vi "Get Available Engine Sim Components.vi"(10 "Register info":T16) -> (2 "Engine Sim Components":T1)   [LabVIEW 2011, in "Engine Sim System Explorer.lvlib"]
uses:
  Engine Sim System Explorer.lvlib
  <userlib>/_FPGA Interface Advanced Tools/FPGA Bitfile Utility/TypeDefs/Scalar Register Set.ctl
  <userlib>/_FPGA Interface Advanced Tools/FPGA Bitfile Utility/TypeDefs/Scalar Register.ctl
  <userlib>/_FPGA Interface Advanced Tools/FPGA Bitfile Utility/TypeDefs/Array Register Set.ctl
  <userlib>/_FPGA Interface Advanced Tools/FPGA Bitfile Utility/TypeDefs/Array Register.ctl
  <userlib>/_FPGA Interface Advanced Tools/FPGA Bitfile Utility/TypeDefs/FIFO Channel Set.ctl
  <userlib>/_FPGA Interface Advanced Tools/FPGA Bitfile Utility/TypeDefs/FIFO Channel.ctl
  TypeDefs/EngineSimComps.ctl
  TypeDefs/APUComp.ctl
  TypeDefs/NTeethComp.ctl
  TypeDefs/FullyCustomComp.ctl
  Shared/FullyCustomCommMode.ctl
  TypeDefs/FullyCustomProfilesComp.ctl
  TypeDefs/ECUEventComp.ctl
  TypeDefs/DataReplayLoopComp.ctl
  TypeDefs/DataReplayComp.ctl
  Engine Simulation Shared.lvlib
  <userlib>/_FPGA Interface Advanced Tools/FPGA Bitfile Utility/FPGA Bitfile Utility.lvlib
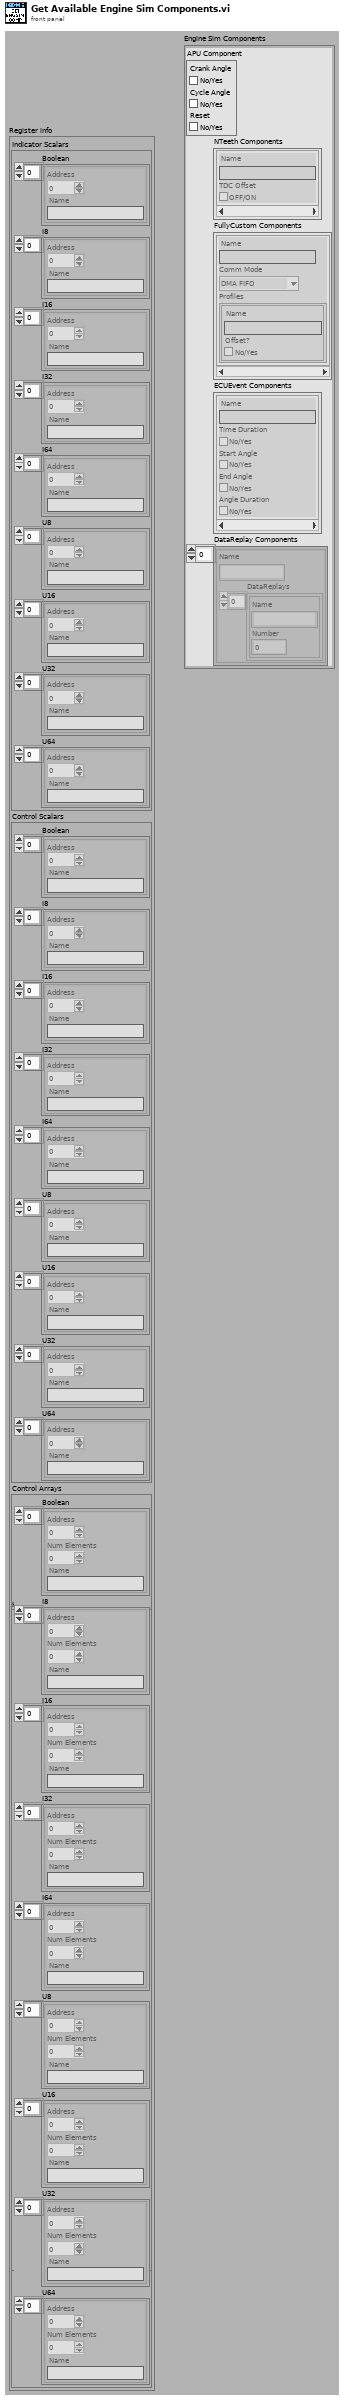
[diagram p1: front panel]
types:
  T1 = typedef "Engine Sim System Explorer.lvlib/EngineSimComps.ctl" = cluster{"APU Component":T2, "NTeeth Components":T3[], "FullyCustom Components":T4[], "ECUEvent Components":T7[], "DataReplay Components":T8[]}
  T2 = typedef "Engine Sim System Explorer.lvlib/APUComp.ctl" = cluster{"Crank Angle":bool, "Cycle Angle":bool, "Reset":bool}
  T3 = typedef "Engine Sim System Explorer.lvlib/NTeethComp.ctl" = cluster{"Name":string, "TDC Offset":bool}
  T4 = typedef "Engine Sim System Explorer.lvlib/FullyCustomComp.ctl" = cluster{"Name":string, "Comm Mode":T5, "Profiles":T6[]}
  T5 = typedef "Engine Simulation Shared.lvlib/FullyCustomCommMode.ctl" = enum16{"DMA FIFO", "FP Data Transfer"}
  T6 = typedef "Engine Sim System Explorer.lvlib/FullyCustomProfilesComp.ctl" = cluster{"Name":string, "Offset?":bool}
  T7 = typedef "Engine Sim System Explorer.lvlib/ECUEventComp.ctl" = cluster{"Name":string, "Time Duration":bool, "Start Angle":bool, "End Angle":bool, "Angle Duration":bool}
  T8 = typedef "Engine Sim System Explorer.lvlib/DataReplayLoopComp.ctl" = cluster{"Name":string, "DataReplays":T9[]}
  T9 = typedef "Engine Sim System Explorer.lvlib/DataReplayComp.ctl" = cluster{"Name":string, "Number":u8}
  T10 = typedef "FPGA Bitfile Utility.lvlib/Scalar Register Set.ctl" = cluster{"Boolean":T11[], "I8":T11[], "I16":T11[], "I32":T11[], "I64":T11[], "U8":T11[], "U16":T11[], "U32":T11[], "U64":T11[]}
  T11 = typedef "FPGA Bitfile Utility.lvlib/Scalar Register.ctl" = cluster{"Address":u32, "Name":string}
  T12 = typedef "FPGA Bitfile Utility.lvlib/Array Register Set.ctl" = cluster{"Boolean":T13[], "I8":T13[], "I16":T13[], "I32":T13[], "I64":T13[], "U8":T13[], "U16":T13[], "U32":T13[], "U64":T13[]}
  T13 = typedef "FPGA Bitfile Utility.lvlib/Array Register.ctl" = cluster{"Address":u32, "Num Elements":u32, "Name":string}
  T14 = typedef "FPGA Bitfile Utility.lvlib/FIFO Channel Set.ctl" = cluster{"Boolean":T15[], "I8":T15[], "I16":T15[], "I32":T15[], "I64":T15[], "U8":T15[], "U16":T15[], "U32":T15[], "U64":T15[]}
  T15 = typedef "FPGA Bitfile Utility.lvlib/FIFO Channel.ctl" = cluster{"Physical Channel":u32, "Name":string}
  T16 = cluster{"Indicator Scalars":T10, "Control Scalars":T10, "Control Arrays":T12, "HostToTarget":T14}
  T17 = cluster{cluster{"Name":string, "Offset":bool}[]}[]
  T18 = typedef "Engine Sim System Explorer.lvlib/FullyCustomRegs.ctl" = cluster{"Num Angles":bool, "Num Profiles":bool, "Angles FIFO":bool, "Data":bool, "Toggle":bool, "LoadComplete":bool, "Profiles":cluster{"First Rising?":bool, "Offset":bool}[]}
  T19 = cluster{"FullyCustomTeeth Names":string[], "FullyCustomTeeths Profile Names":cluster{"FullyCustomTeeth Profile Names":string[]}[], "FullyCustomTeeth Regs":T18[]}
  T20 = typedef "Engine Sim System Explorer.lvlib/ECUEventRegs.ctl" = cluster{"Time Duration":bool, "Start Angle":bool, "End Angle":bool, "Angle Duration":bool}
  T21 = cluster{"ECUEvent Names":string[], "ECUEvent Regs":T20[]}
  T22 = typedef "Engine Sim System Explorer.lvlib/NTeethRegs.ctl" = cluster{"Deg High Pulse":bool, "Deg Low Pulse":bool, "TDC High?":bool, "Num Teeth Miss":bool, "Miss Teeth Offset":bool, "TDC Offset":bool}
  T23 = cluster{"NTeeth Names":string[], "NTeeth Regs":T22[]}
  T24 = cluster{"FullyCustomTeeth Profile Names":string[]}[]
  T25 = cluster{"FullyCustomTeeth Profile Names":string[]}
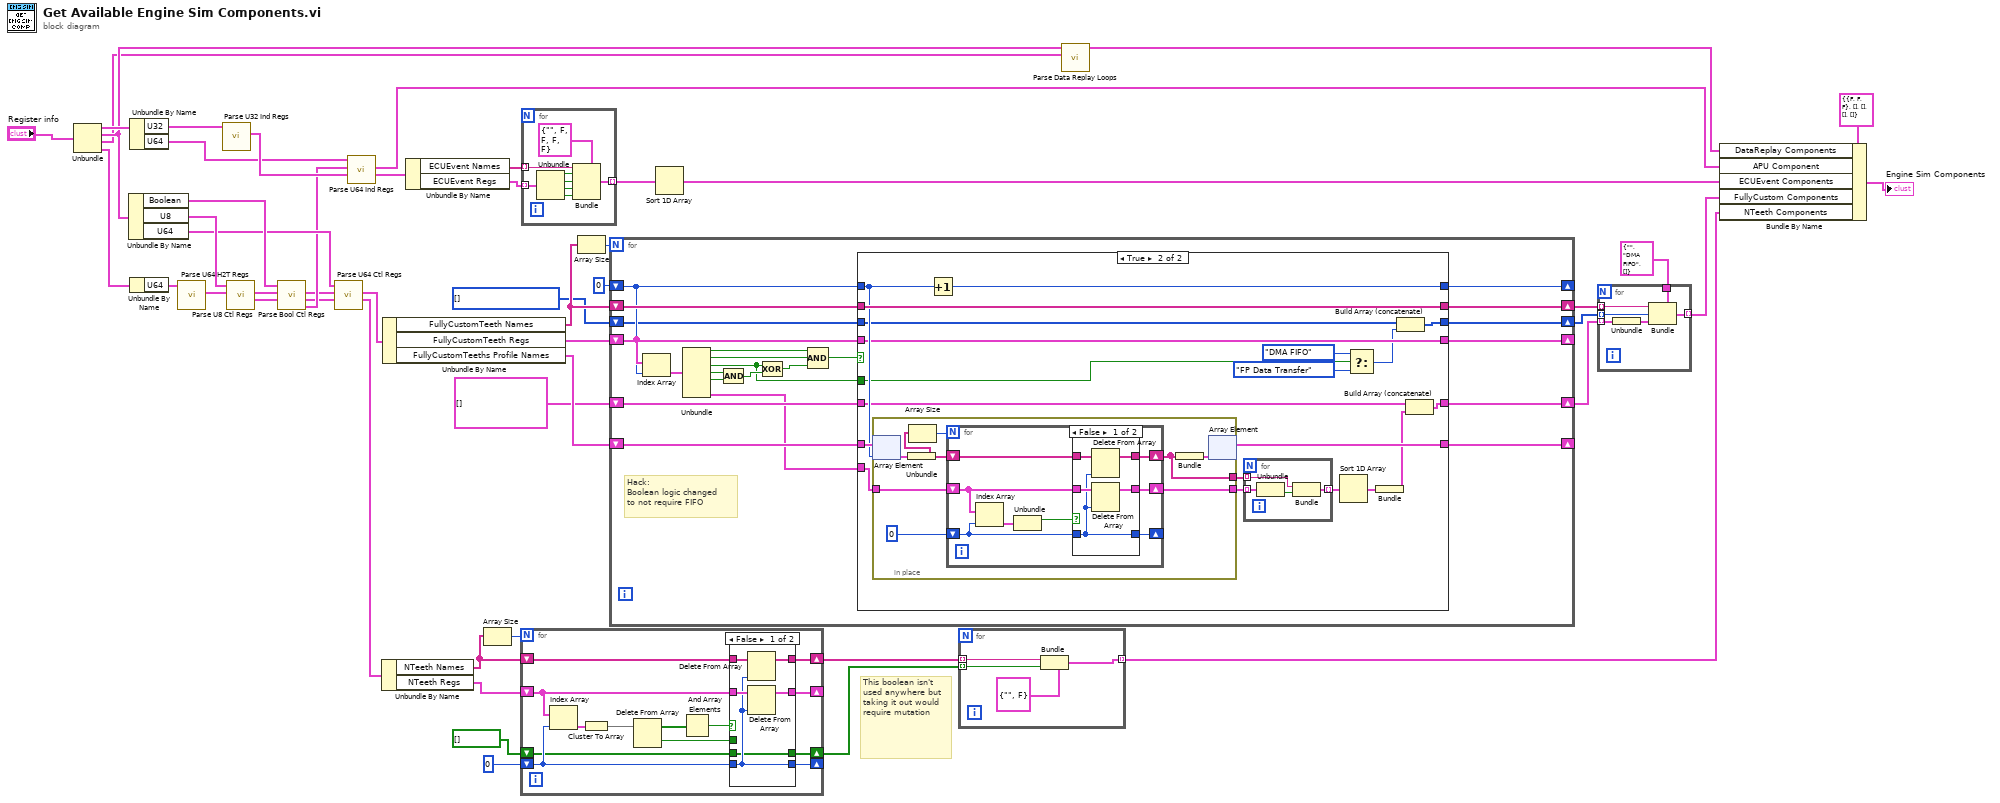
[diagram p0: block diagram]
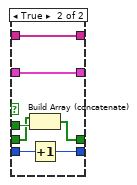
[diagram p2: hidden frame]
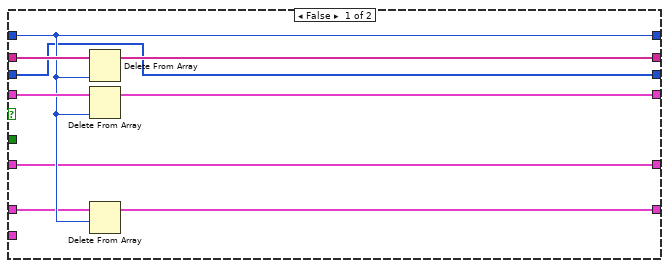
[diagram p3: hidden frame]
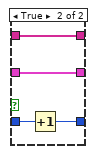
[diagram p4: hidden frame]
diagram:
  w11 = T5[] [] items=["DMA FIFO", "FP Data Transfer"]
  # "This boolean isn't used anywhere but taking it out would require mutation"
  n1 = Unbundle("Register info") -> ("Indicator Scalars"=w7:T10, "Control Scalars"=w4:T10, "Control Arrays"=w1:T12, "HostToTarget"=w2:T14)
  n2 = Unbundle By Name(w4) -> ("Boolean"=w29:T11[], "U8"=w43:T11[], "U64"=w27:T11[])
  n3 = Unbundle By Name(w7) -> ("U32"=w48:T11[], "U64"=w36:T11[])
  n4 = Unbundle By Name(w2) -> ("U64"=w44:T15[])
  n5 = call "Parse U64 H2T Regs.vi"("U64"=w44) -> ("FullyCustomTeeths Out"=w12:T19)  [unwired: 10 in]
  n6 = call "Parse U32 Ind Regs.vi"("U32 Registers"=w48) -> ("ECUEvents Out"=w37:T21)  [unwired: 10 in]
  n7 = call "Parse U8 Ctl Regs.vi"("FullyCustomTeeths In"=w12, "U8"=w43) -> ("NTeeths Out"=w28:T23, "FullyCustomTeeths In"=w9:T19)  [unwired: 8 in]
  n8 = call "Parse Bool Ctl Regs.vi"("NTeeths In"=w28, "FullyCustomTeeths In"=w9, "Boolean"=w29) -> ("APU Registers Out"=w15:T2, "NTeeths Out"=w13:T23, "FullyCustomTeeths In"=w8:T19)  [unwired: 6 in]
  n9 = call "Parse U64 Ctl Regs.vi"("NTeeths In"=w13, "FullyCustomTeeths In"=w8, "U64"=w27) -> ("NTeeths Out"=w22:T23, "FullyCustomTeeths In"=w26:T19)  [unwired: 7 in]
  n10 = call "Parse U64 Ind Regs.vi"("ECUEvents In"=w37, "APU Registers In"=w15, "U64"=w36) -> ("ECUEvents Out"=w35:T21, "APU Registers Out"=w32:T2)  [unwired: 7 in]
  n11 = Unbundle By Name(w22) -> ("NTeeth Names"=w5:string[], "NTeeth Regs"=w21:T22[])
  n12 = Unbundle By Name(w26) -> ("FullyCustomTeeth Names"=w31:string[], "FullyCustomTeeth Regs"=w30:T18[], "FullyCustomTeeths Profile Names"=w25:T24)
  n13 = Unbundle By Name(w35) -> ("ECUEvent Names"=w34:string[], "ECUEvent Regs"=w33:T20[])
  n14 = Array Size(array=w5) -> (size(s)=w19:i32)
  n15 = for {
    N: w19 -> [_]
    shift-right: [w60] -> _
    shift-left: w21 -> [w61]
    shift-right: [w58] -> w18
    shift-left: w5 -> [w59]
    shift-right: [w57] -> _
    shift-left: 0 -> [w56]
    shift-right: [w51] -> w14
    shift-left: bool[] [] -> [w50]
    n16 = Index Array(array=w61, index=w56) -> (element=w62:T22)
    n17 = Cluster To Array(cluster=w62) -> (array=w54:bool[])
    n18 = Delete From Array(array=w54) -> (deleted portion=w52:bool, array with subset deleted=w53:bool[])  [unwired: 2 in]
    n19 = And Array Elements(Boolean array=w53) -> (logical AND=w55:bool)
    n20 = case shown="False" w55 {
      tunnel: w61 -> [w68 w74]
      tunnel: [w67 w74] -> w60
      tunnel: w59 -> [w66 w75]
      tunnel: [w65 w75] -> w58
      tunnel: [w64 w73] -> w57
      tunnel: w56 -> [w64 w72]
      tunnel: w52 -> [_ w71]
      tunnel: [w63 w70] -> w51
      tunnel: w50 -> [w63 w69]
      frame False {
        n21 = Delete From Array(array=w66, index=w64) -> (array with subset deleted=w65:string[])  [unwired: 1 in, 1 out]
        n22 = Delete From Array(array=w68, index=w64) -> (array with subset deleted=w67:T22[])  [unwired: 1 in, 1 out]
      }
      frame True {
        n23 = Build Array (concatenate)(w69, w71) -> (w70:bool[])
        n24 = Increment(x=w72) -> (x+1=w73:i32)
      }
    }
  }
  n25 = for {
    tunnel: w34 -> [w83] mode=indexing
    tunnel: w33 -> [w82] mode=indexing
    tunnel: [w77] -> w46 mode=indexing
    n26 = Unbundle(w82) -> ("Time Duration"=w81:bool, "Start Angle"=w80:bool, "End Angle"=w79:bool, "Angle Duration"=w78:bool)
    n27 = Bundle(cluster=T7 {"Name"="", "Time Duration"=FALSE, "Start Angle"=FALSE, "End Angle"=FALSE, "Angle Duration"=FALSE} ("ECU Event Component"), "Name"=w83, "Time Duration"=w81, "Start Angle"=w80, "End Angle"=w79, "Angle Duration"=w78) -> (w77:T7)
  }
  n28 = Array Size(array=w31) -> (size(s)=w41:i32)
  n29 = for {
    N: w41 -> [_]
    shift-right: [w101] -> _
    shift-left: w30 -> [w102]
    shift-right: [w99] -> w40
    shift-left: w31 -> [w100]
    shift-right: [w98] -> _
    shift-left: 0 -> [w97]
    shift-right: [w95] -> _
    shift-left: w25 -> [w96]
    shift-right: [w93] -> w23
    shift-left: T17 [] -> [w92]
    shift-right: [w84] -> w10
    shift-left: w11 -> [w85]
    # "Hack: \nBoolean logic changed\nto not require FIFO"
    n30 = Index Array(array=w102, index=w97) -> (element=w94:T18)
    n31 = Unbundle(w94) -> ("Num Angles"=w104:bool, "Num Profiles"=w105:bool, "Angles FIFO"=w86:bool, "Data"=w89:bool, "Toggle"=w90:bool, "Profiles"=w91:cluster{"First Rising?":bool, "Offset":bool}[])  [unwired: 1 out]
    n32 = Compound Arithmetic op=AND(w89, w90) -> (w88:bool)
    n33 = Compound Arithmetic op=XOR(w86, w88) -> (w87:bool)
    n34 = Compound Arithmetic op=AND(w104, w105, w87) -> (w103:bool)
    n35 = case shown="True" w103 {
      tunnel: w102 -> [w114 w128]
      tunnel: [w113 w128] -> w101
      tunnel: w100 -> [w112 w134]
      tunnel: [w111 w134] -> w99
      tunnel: [w110 w133] -> w98
      tunnel: w97 -> [w110 w129]
      tunnel: w96 -> [w109 w131]
      tunnel: [w108 w130] -> w95
      tunnel: w91 -> [_ w132]
      tunnel: [w107 w127] -> w93
      tunnel: w92 -> [w107 w126]
      tunnel: w86 -> [_ w118]
      tunnel: w85 -> [w106 w117]
      tunnel: [w106 w115] -> w84
      frame False {
        n36 = Delete From Array(array=w112, index=w110) -> (array with subset deleted=w111:string[])  [unwired: 1 in, 1 out]
        n37 = Delete From Array(array=w114, index=w110) -> (array with subset deleted=w113:T18[])  [unwired: 1 in, 1 out]
        n38 = Delete From Array(array=w109, length=w110) -> (array with subset deleted=w108:T24)  [unwired: 1 in, 1 out]
      }
      frame True {
        n39 = in-place {
          in-place-border: w132 -> [w146]
          in-place-border: [w142] -> w125
          in-place-border: [w141] -> w124
          n40 = in-place-array #1(w131, w129) -> (w144:T25)
          n41 = Unbundle(w144) -> ("FullyCustomTeeth Profile Names"=w140:string[])
          n42 = Array Size(array=w140) -> (size(s)=w139:i32)
          n43 = for {
            N: w139 -> [_]
            shift-right: [w152] -> w142
            shift-left: w146 -> [w153]
            shift-right: [w150] -> w141
            shift-left: w140 -> [w151]
            shift-right: [w149] -> _
            shift-left: 0 -> [w148]
            n44 = Index Array(array=w153, index=w148) -> (element=w154:cluster{"First Rising?":bool, "Offset":bool})
            n45 = Unbundle(w154) -> ("First Rising?"=w147:bool)  [unwired: 1 out]
            n46 = case shown="False" w147 {
              tunnel: w153 -> [w159 w162]
              tunnel: [w158 w162] -> w152
              tunnel: w151 -> [w157 w163]
              tunnel: [w156 w163] -> w150
              tunnel: [w155 w161] -> w149
              tunnel: w148 -> [w155 w160]
              frame False {
                n47 = Delete From Array(array=w157, index=w155) -> (array with subset deleted=w156:string[])  [unwired: 1 in, 1 out]
                n48 = Delete From Array(array=w159, index=w155) -> (array with subset deleted=w158:cluster{"First Rising?":bool, "Offset":bool}[])  [unwired: 1 in, 1 out]
              }
              frame True {
                n49 = Increment(x=w160) -> (x+1=w161:i32)
              }
            }
          }
          n50 = Bundle("FullyCustomTeeth Profile Names"=w141) -> (w143:T25)  [unwired: 1 in]
          n51 = in-place-array #1(w143) -> (w130:T24)  [unwired: 1 out]
        }
        n52 = Increment(x=w129) -> (x+1=w133:i32)
        n53 = for {
          tunnel: w125 -> [w138] mode=indexing
          tunnel: w124 -> [w136] mode=indexing
          tunnel: [w135] -> w123 mode=indexing
          n54 = Unbundle(w138) -> ("Offset"=w137:bool)  [unwired: 1 out]
          n55 = Bundle("Name"=w136, "Offset"=w137) -> (w135:cluster{"Name":string, "Offset":bool})  [unwired: 1 in]
        }
        n56 = Sort 1D Array(array=w123) -> (sorted array=w121:cluster{"Name":string, "Offset":bool}[])
        n57 = Select(t=FullyCustomCommMode."DMA FIFO" ("Comm Mode"), s=w118, f=FullyCustomCommMode."FP Data Transfer" ("Comm Mode")) -> (s? t:f=w116:T5)
        n58 = Bundle(w121) -> (w122:cluster{cluster{"Name":string, "Offset":bool}[]})  [unwired: 1 in]
        n59 = Build Array (concatenate)(w117, w116) -> (w115:T5[])
        n60 = Build Array (concatenate)(w126, w122) -> (w127:T17)
      }
    }
  }
  n61 = Sort 1D Array(array=w46) -> (sorted array=w16:T7[])
  n62 = for {
    tunnel: w18 -> [w167] mode=indexing
    tunnel: [w166] -> w17 mode=indexing
    tunnel: w14 -> [w165] mode=indexing
    n63 = Bundle(cluster=T3 {"Name"="", "TDC Offset"=FALSE} ("NTeeth Component"), "Name"=w167, "TDC Offset"=w165) -> (w166:T3)
  }
  n64 = call "Parse Data Replay Loops.vi"("Control Arrays"=w1, "Control Scalars"=w4) -> ("DataReplay Loops"=w3:T8[])  [unwired: 9 in]
  n65 = for {
    tunnel: w40 -> [w173] mode=indexing
    tunnel: [w172] -> w38 mode=indexing
    tunnel: T4 {"Name"="", "Comm Mode"=enum."DMA FIFO", "Profiles"=[]} ("FullyCustom Component") -> [w171]
    tunnel: w23 -> [w170] mode=indexing
    tunnel: w10 -> [w168] mode=indexing
    n66 = Unbundle(w170) -> (w169:cluster{"Name":string, "Offset":bool}[])
    n67 = Bundle(cluster=w171, "Name"=w173, "Comm Mode"=w168, "Profiles"=w169) -> (w172:T4)
  }
  n68 = Bundle By Name(cluster=T1 {"APU Component"={"Crank Angle"=FALSE, "Cycle Angle"=FALSE, "Reset"=FALSE}, "NTeeth Components"=[], "FullyCustom Components"=[], "ECUEvent Components"=[], "DataReplay Components"=[]} ("Engine Sim Components"), "DataReplay Components"=w3, "APU Component"=w32, "ECUEvent Components"=w16, "FullyCustom Components"=w38, "NTeeth Components"=w17) -> (→"Engine Sim Components":T1)
